vi "HK Channel CVT Add Value.vi"(7 "CVT Settings":T3 {"Max Age" format="%<%H:%M:%S>t"}, 9 "Timestamp":timestamp, 10 "New Value":dbl, 11 "Current Value":T1) -> (2 "time stamp":timestamp, 3 "Current Value out":T1)   [LabVIEW 2019, in "HK Table.lvclass"]
uses:
  HK Table.lvclass
  HK Current Value Table Element.ctl
  HK Alarms/HK Alarm enum Status.ctl
  HK Current Value Table Settings.ctl
  HK Item/HK Item.lvclass
panel:
  out "recent times":timestamp[](array[timestamp])
  out "recent values":dbl[](array[numeric])
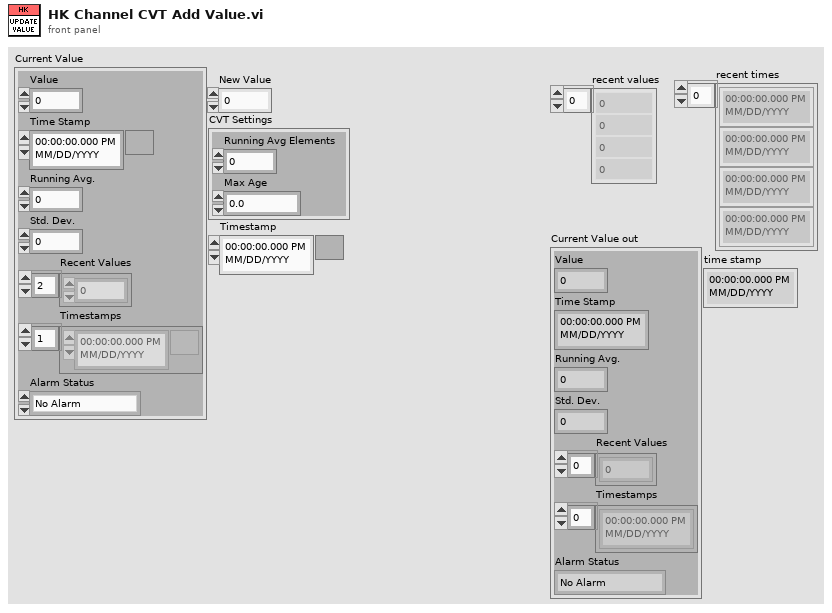
[diagram p1: front panel]
types:
  T1 = typedef "HK Table.lvclass/HK Current Value Table Element.ctl" = cluster{"Value":dbl, "Time Stamp":timestamp, "Running Avg.":dbl, "Std. Dev.":dbl, "Recent Values":dbl[], "Timestamps":timestamp[], "Alarm Status":T2}
  T2 = typedef "HK Item.lvclass/HK Alarm enum Status.ctl" = enum16{"No Alarm", "Red Low", "Red High", "Yellow Low", "Yellow High"}
  T3 = typedef "HK Table.lvclass/HK Current Value Table Settings.ctl" = cluster{"Running Avg Elements":i32, "Max Age":dbl}
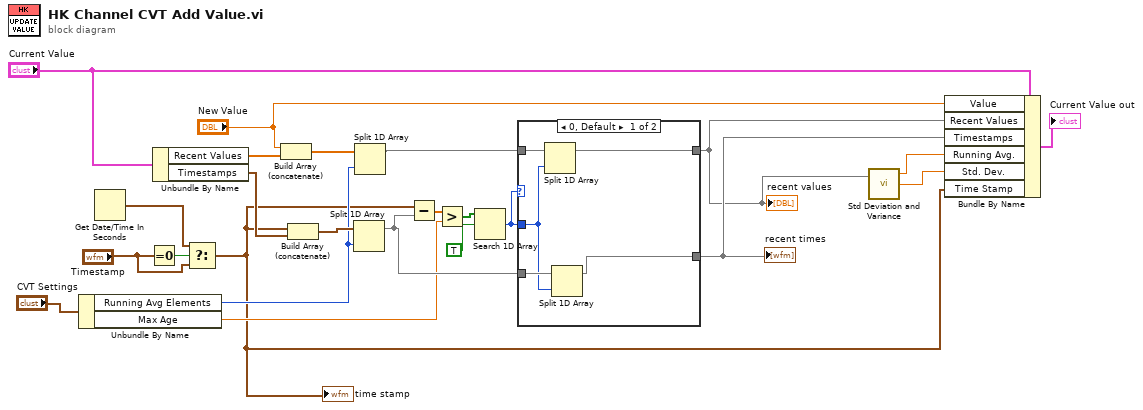
[diagram p0: block diagram]
diagram:
  n1 = Unbundle By Name("CVT Settings") -> ("Running Avg Elements"=w19:i32, "Max Age"=w12:dbl)
  n2 = Get Date/Time In Seconds() -> (seconds since 1Jan1904=w3:timestamp)
  n3 = Equal To 0?(x="Timestamp") -> (x = 0?=w4:bool)
  n4 = Unbundle By Name("Current Value") -> ("Recent Values"=w24:dbl[], "Timestamps"=w21:timestamp[])
  n5 = Select(t=w3, s=w4, f="Timestamp") -> (s? t:f=w1:timestamp)
  "time stamp" <- w1
  n6 = Build Array (concatenate)("New Value", w24) -> (w23:dbl[])
  n7 = Build Array (concatenate)(w1, w21) -> (w20:timestamp[])
  n8 = Split 1D Array(array=w20, index=w19) -> (first subarray=w14:timestamp[])  [unwired: 1 out]
  n9 = Split 1D Array(array=w23, index=w19) -> (first subarray=w15:dbl[])  [unwired: 1 out]
  n10 = Subtract(x=w1, y=w14) -> (x-y=w13:dbl[])
  n11 = Greater?(x=w13, y=w12) -> (0:w11:bool[])
  n12 = Search 1D Array(1D array=w11, element=TRUE) -> (index of element=w9:i32)  [unwired: 1 in]
  n13 = case shown="0, Default" w9 {
    tunnel: [w29 w31] -> w7
    tunnel: [w28 w30] -> w8
    tunnel: w15 -> [w27 w31]
    tunnel: w14 -> [w26 w30]
    tunnel: w9 -> [w25 _]
    frame 0, Default {
      n14 = Split 1D Array(array=w27, index=w25) -> (first subarray=w29:dbl[])  [unwired: 1 out]
      n15 = Split 1D Array(array=w26, index=w25) -> (first subarray=w28:timestamp[])  [unwired: 1 out]
    }
    frame -1 {
    }
  }
  "recent times" <- w8
  "recent values" <- w7
  n16 = call <vilib>:"Std Deviation and Variance.vi"("X"=w7) -> ("mean"=w6:dbl, "standard deviation"=w5:dbl)  [unwired: 1 in, 1 out]
  n17 = Bundle By Name(cluster="Current Value", "Value"="New Value", "Recent Values"=w7, "Timestamps"=w8, "Running Avg."=w6, "Std. Dev."=w5, "Time Stamp"=w1) -> (→"Current Value out":T1)
